vi "Core Wrapper.vi"(0 "Controller in":refnum<class "Controller.lvclass">, 5 "error in (no error)":errorcluster) -> (14 "Controller out":refnum<class "Controller.lvclass">, 19 "error out":errorcluster)   [LabVIEW 2014, in "Controller.lvlib" / "Controller.lvclass"]
doc: "This is a wrapper for controller functionality intended to run parallel to the Actor Core. It is not reentrant and thus allows the user to debug this portion of the actor."
uses:
  Controller.lvclass
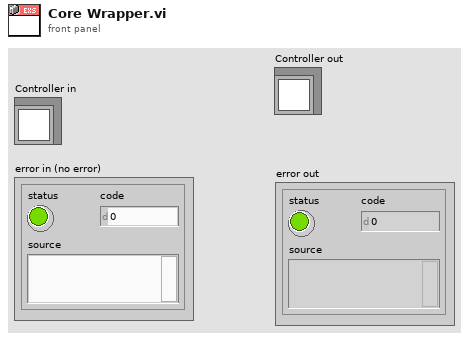
[diagram p1: front panel]
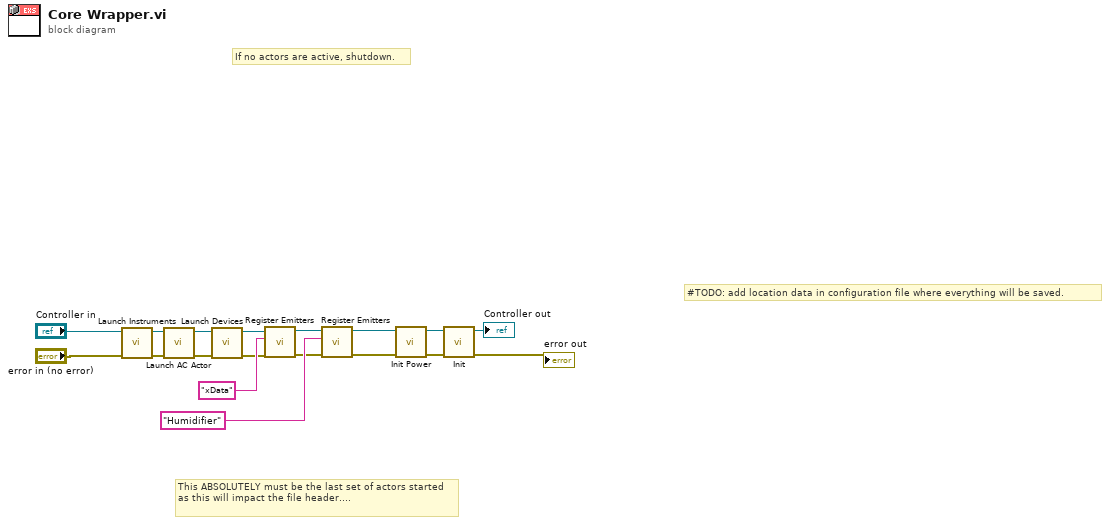
[diagram p0: block diagram]
diagram:
  # "If no actors are active, shutdown."
  # "This ABSOLUTELY must be the last set of actors started as this will impact the file header...."
  # "#TODO: add location data in configuration file where everything will be saved."
  n1 = call "Launch Instruments.vi"("error in"="error in (no error)", "Controller in"="Controller in") -> ("error out"=w7:errorcluster, "Controller out"=w6:refnum<class "Controller.lvclass">)  [unwired: 8 in]
  n2 = call "Launch AC Actor.vi"("error in"=w7, "Controller in"=w6) -> ("error out"=w13:errorcluster, "Controller out"=w3:refnum<class "Controller.lvclass">)  [unwired: 8 in]
  n3 = call "Launch Devices.vi"("error in"=w13, "Controller In"=w3) -> ("error out"=w9:errorcluster, "Controller Out"=w8:refnum<class "Controller.lvclass">)  [unwired: 8 in]
  n4 = call "Register Emitters.vi"("error in"=w9, "Emitter"="xData", "Controller in"=w8) -> ("error out"=w16:errorcluster, "Controller out"=w14:refnum<class "Controller.lvclass">)  [unwired: 7 in]
  n5 = call "Register Emitters.vi"("error in"=w16, "Emitter"="Humidifier", "Controller in"=w14) -> ("error out"=w17:errorcluster, "Controller out"=w15:refnum<class "Controller.lvclass">)  [unwired: 7 in]
  n6 = call "Init Power.vi"("error in"=w17, "Controller in"=w15) -> ("error out"=w12:errorcluster, "Controller out"=w11:refnum<class "Controller.lvclass">)  [unwired: 8 in]
  n7 = call "Init.vi"("error in"=w12, "Controller in"=w11) -> ("error out"=→"error out":errorcluster, "Controller out"=→"Controller out":refnum<class "Controller.lvclass">)  [unwired: 8 in]
